vi "Make Full Factorial Experiment.vi"(11 "Array of Array Settings":T1(array[cluster])) -> (3 "Full Factorial Design":string[][](array[string]))   [LabVIEW 2010]
panel:
  out "product":dbl
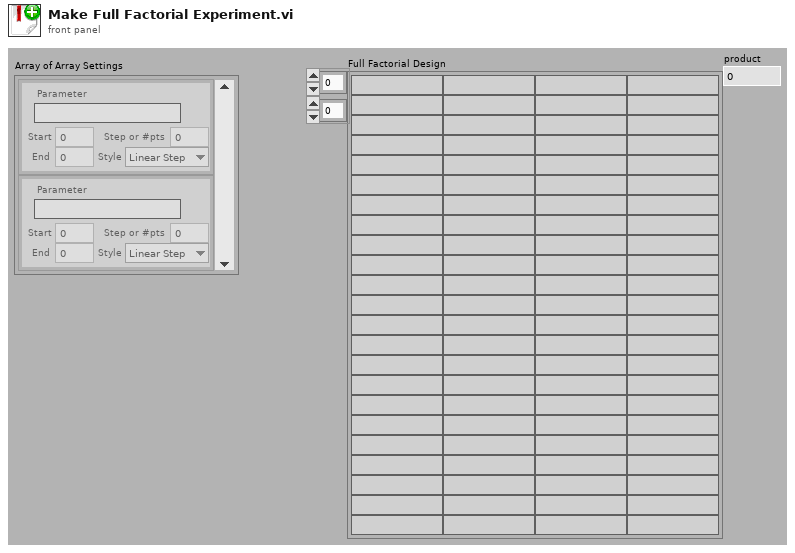
[diagram p1: front panel]
types:
  T1 = cluster{"Start":dbl, "End":dbl, "Step or #pts":dbl, "Style":enum16{"Linear Step", "Linear Pts", "Log Pts"}, "Parameter":string}[]
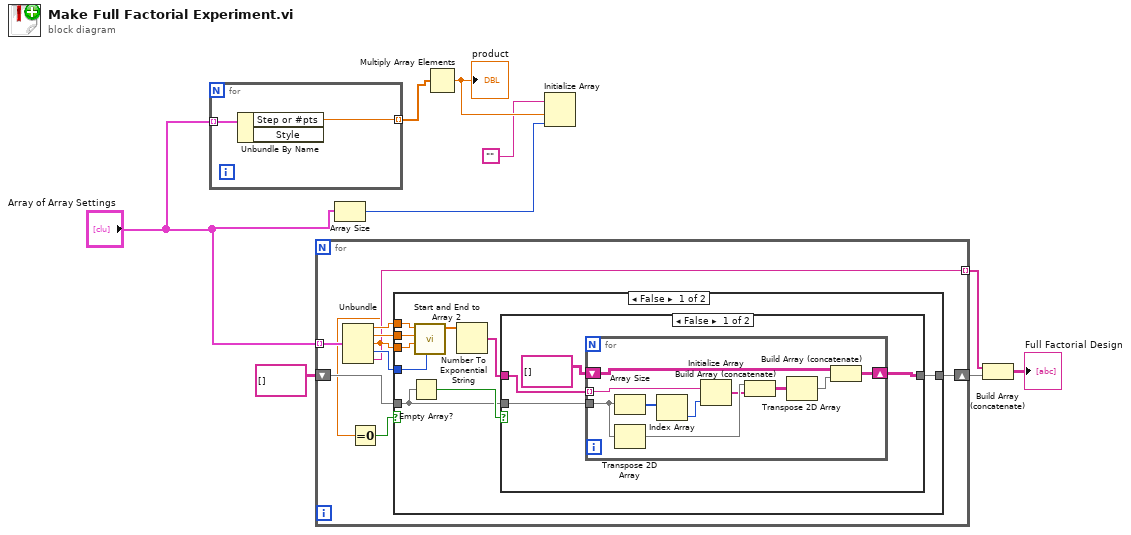
[diagram p0: block diagram]
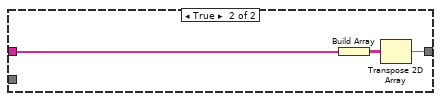
[diagram p2: hidden frame]
diagram:
  n1 = for {
    tunnel: "Array of Array Settings" -> [w11] mode=indexing
    tunnel: [w10] -> w7 mode=indexing
    n2 = Unbundle By Name(w11) -> ("Step or #pts"=w10:dbl)  [unwired: 1 out]
  }
  n3 = for {
    tunnel: "Array of Array Settings" -> [w20] mode=indexing
    tunnel: [w16] -> w8 mode=indexing
    shift-right: [w15] -> w6
    shift-left: string[][] [] -> [w14]
    n4 = Unbundle(w20) -> ("Start"=w19:dbl, "End"=w18:dbl, "Step or #pts"=w13:dbl, "Style"=w17:enum16{"Linear Step", "Linear Pts", "Log Pts"}, "Parameter"=w16:string)
    n5 = Equal To 0?(x=w13) -> (x = 0?=w12:bool)
    n6 = case shown="False" w12 {
      tunnel: w19 -> [w29 _]
      tunnel: w18 -> [w28 _]
      tunnel: w13 -> [w27 _]
      tunnel: w17 -> [w26 _]
      tunnel: [w24 w47] -> w15
      tunnel: w14 -> [w21 w47]
      frame False {
        n7 = Empty Array?(array=w21) -> (empty?=w23:bool)
        n8 = call "Start and End to Array 2.vi"("Sweep Style"=w26, "Step or # Pts"=w27, "End"=w28, "Start"=w29) -> ("Array"=w25:dbl[])  [unwired: 7 in]
        n9 = Number To Exponential String(number=w25) -> (E-format string=w22:string[])  [unwired: 3 in]
        n10 = case shown="False" w23 {
          tunnel: [w33 w44] -> w24
          tunnel: w22 -> [w31 w45]
          tunnel: w21 -> [w30 _]
          frame False {
            n11 = for {
              tunnel: w31 -> [w43] mode=indexing
              shift-right: [w35] -> w33
              shift-left: string[][] [] -> [w34]
              tunnel: w30 -> [w40]
              n12 = Array Size(array=w40) -> (size(s)=w42:i32[])
              n13 = Transpose 2D Array(2D array=w40) -> (transposed array=w39:string[][])
              n14 = Index Array(array=w42) -> (element=w41:i32)  [unwired: 1 in]
              n15 = Initialize Array(w43, w41) -> (w38:string[])
              n16 = Build Array (concatenate)(w39, w38) -> (w37:string[][])
              n17 = Transpose 2D Array(2D array=w37) -> (transposed array=w36:string[][])
              n18 = Build Array (concatenate)(w34, w36) -> (w35:string[][])
            }
          }
          frame True {
            n19 = Build Array(w45) -> (w46:string[][])
            n20 = Transpose 2D Array(2D array=w46) -> (transposed array=w44:string[][])
          }
        }
      }
      frame True {
      }
    }
  }
  n21 = Array Size(array="Array of Array Settings") -> (size(s)=w3:i32)
  n22 = Multiply Array Elements(1:w7) -> (0:w5:dbl)
  "product" <- w5
  n23 = Initialize Array("", w5, w3) -> ()  [unwired: 1 out]
  n24 = Build Array (concatenate)(w8, w6) -> (→"Full Factorial Design":string[][])
